vi "LogGrapher.vi"() -> ()   [LabVIEW 2016]
uses:
  <vilib>/regexp/Match Regular Expression.xnode
panel:
  in  "indexes":T1={"angle"=9, "left encoder"=12, "right encoder"=13}
  in  "PlaySpeed":dbl(ring)=1.0 items=["x8"=8.0, "x4"=4.0, "x2"=2.0, "x1"=1.0, "x1/2"=0.5]
  in  "Slide":dbl(slide) scale=0.0..150.0
  out "Robot Tracker":cluster{dbl, dbl}[](graph)
  in  "Play/Pause":enum32{"Play", "Pause"}(radio)=enum."Pause"
  out "Legend":string
  out "Log Grapher":cluster{dbl[], dbl[]}[](graph)
  in  "Log Columns":cluster{"Show":bool, "Data":string}[](array[cluster])
  in  "Column of Time":u32
  in  "Row of Headers":u32=4
  in  "1st Row of Data":u32=5
  in  "Log File Path":path
  # "Enter -1 if not applicable."
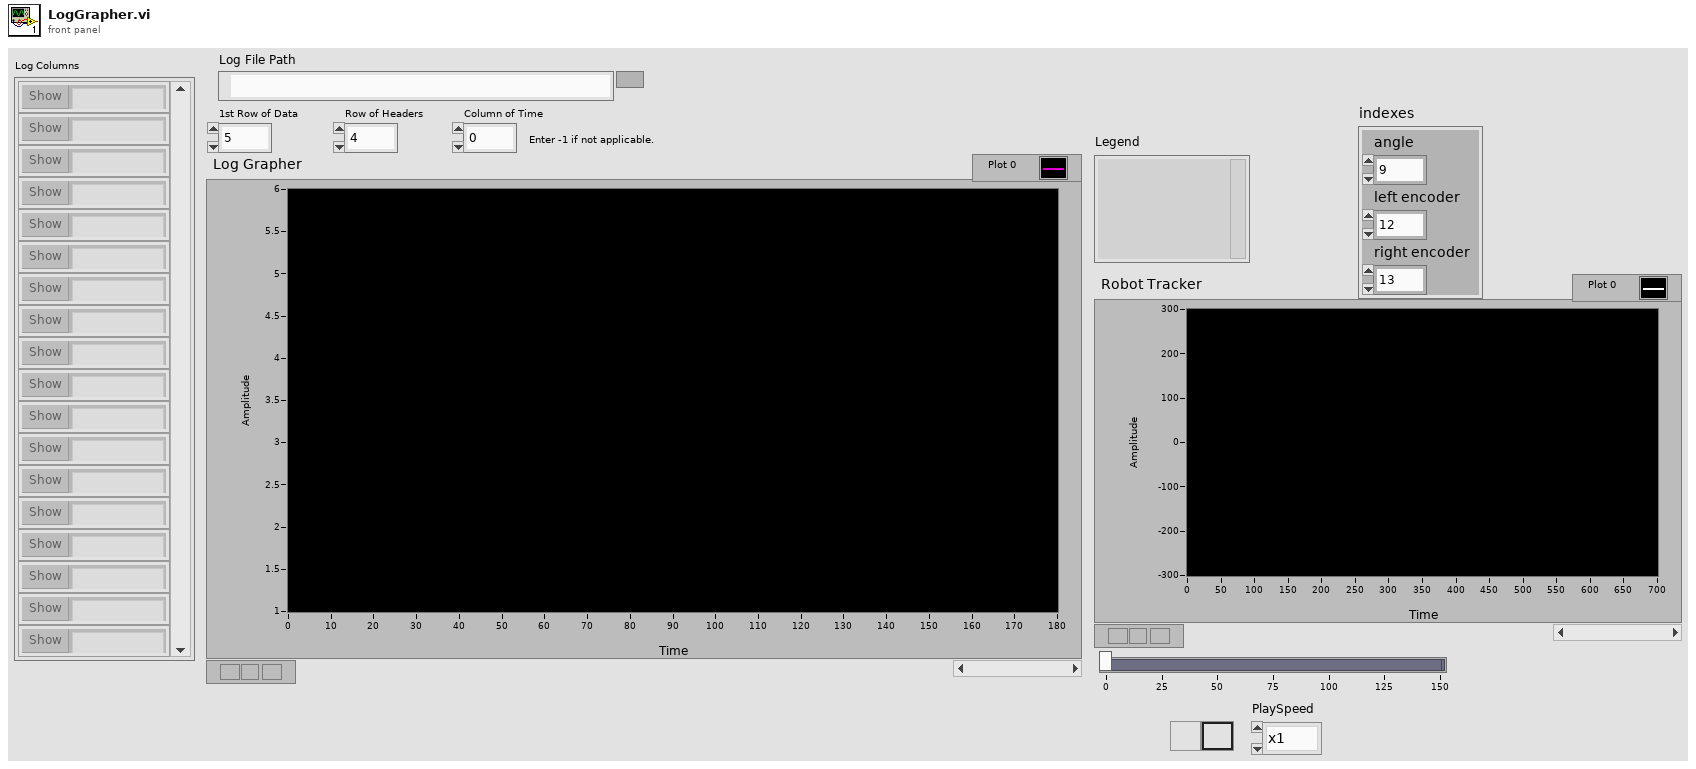
[diagram p1: front panel]
types:
  T1 = cluster{"angle":i32, "left encoder":i32, "right encoder":i32}
  T2 = cluster{"time":i32, "angle":dbl, "left dist":dbl, "right dist":dbl}
  T3 = typedef "LVRangeTypeDef.ctl" = cluster{"Minimum":dbl, "Maximum":dbl, "Increment":dbl, "Minor Increment":dbl, "Start":dbl}
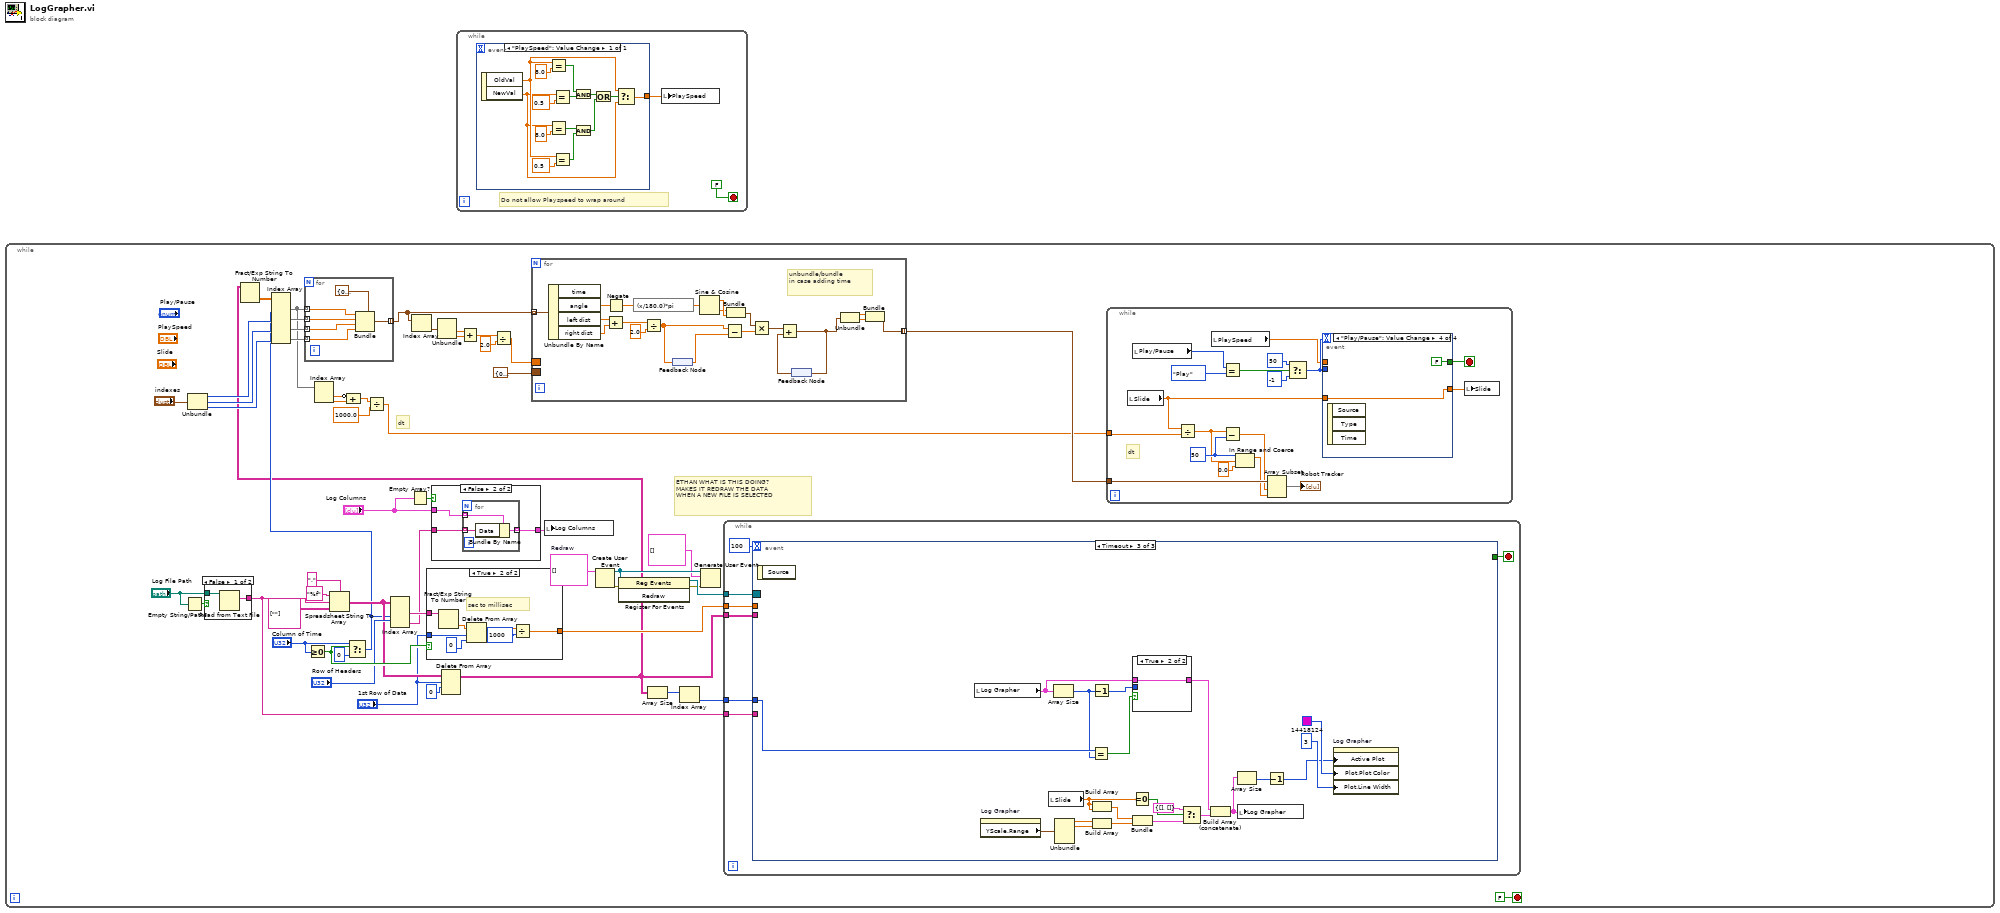
[diagram p0: block diagram]
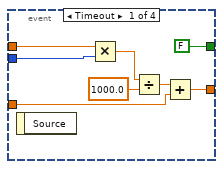
[diagram p2: hidden frame]
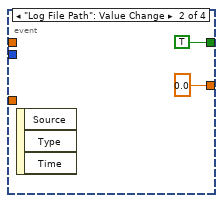
[diagram p3: hidden frame]
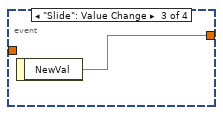
[diagram p4: hidden frame]
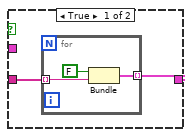
[diagram p5: hidden frame]
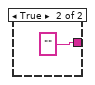
[diagram p6: hidden frame]
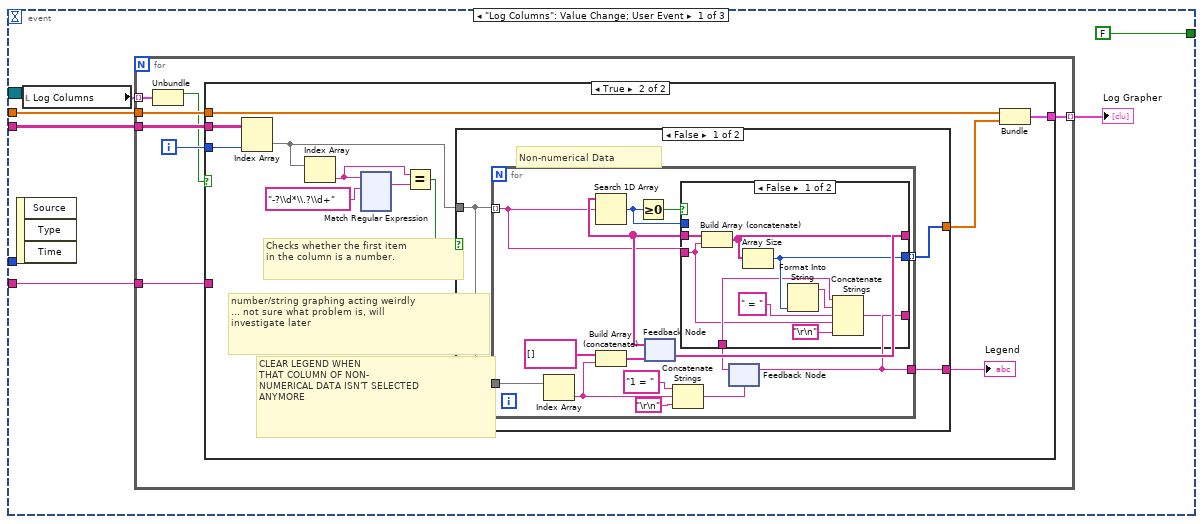
[diagram p7: hidden frame]
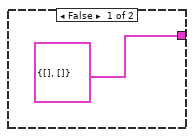
[diagram p8: hidden frame]
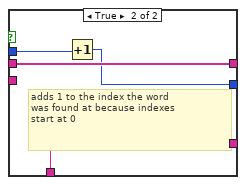
[diagram p9: hidden frame]
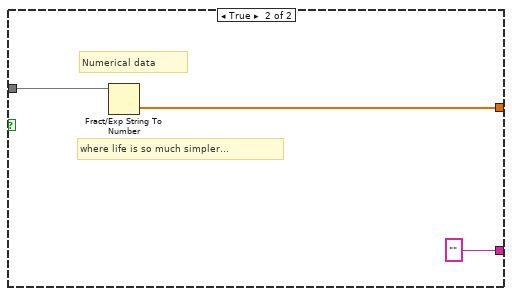
[diagram p10: hidden frame]
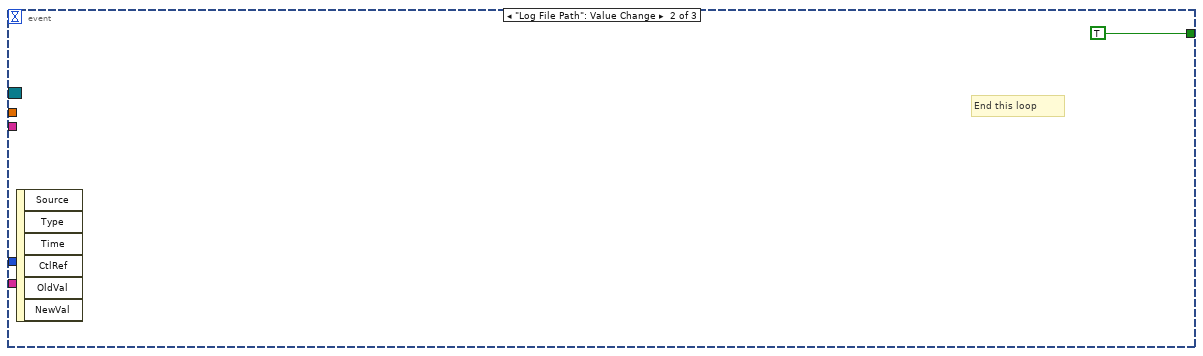
[diagram p11: hidden frame]
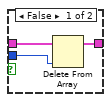
[diagram p12: hidden frame]
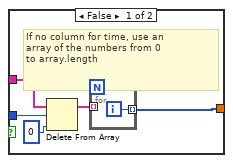
[diagram p13: hidden frame]
diagram:
  n1 = while {
    stop <- FALSE stop-if-true
    w34 = cluster{"Show":bool, "Data":string}[] []  # Redraw
    # "dt"
    # "ETHAN WHAT IS THIS DOING?\nMAKES IT REDRAW THE DATA\nWHEN A NEW FILE IS SELECTED"
    n2 = Empty String/Path?(string/path="Log File Path") -> (empty?=w41:bool)
    n3 = Unbundle("indexes") -> ("angle"=w13:i32, "left encoder"=w12:i32, "right encoder"=w11:i32)
    n4 = case shown="False" w41 {
      tunnel: [w123 ""] -> w28
      tunnel: "Log File Path" -> [w122 _]
      frame False {
        n5 = Read from Text File(file (use dialog)=w122) -> (text=w123:string)  [unwired: 3 in, 3 out]
      }
      frame True {
      }
    }
    n6 = Greater Or Equal To 0?(x="Column of Time") -> (x >= 0?=w47:bool)
    n7 = Spreadsheet String To Array(delimiter (Tab)=",", format string="%f", spreadsheet string=w28, array type (2D Dbl)=string[][] [[""]]) -> (array=w43:string[][])
    n8 = Select(t="Column of Time", s=w47, f=u32 0) -> (s? t:f=w10:u32)
    n9 = Index Array(array=w43, index (col) #1=w10, index (row) #2="Row of Headers") -> (element #1=w50:string[], element #2=w39:string[])  [unwired: 2 in]
    n10 = Empty Array?(array="Log Columns") -> (empty?=w38:bool)
    n11 = case shown="True" w47 {
      tunnel: [w335 w341] -> w36
      tunnel: "1st Row of Data" -> [w332 w340]
      tunnel: w50 -> [w333 w339]
      frame False {
        # "If no column for time, use an\narray of the numbers from 0 \nto array.length"
        n12 = Delete From Array(array=w333, length=w332, index=0) -> (array with subset deleted=w331:string[])  [unwired: 1 out]
        n13 = for {
          tunnel: [w336] -> w335 mode=indexing
          tunnel: w331 -> [_] mode=indexing
          i -> [w336]
        }
      }
      frame True {
        # "sec to millisec"
        n14 = Fract/Exp String To Number(string=w339) -> (number=w338:dbl[])  [unwired: 3 in, 1 out]
        n15 = Delete From Array(array=w338, length=w340, index=0) -> (array with subset deleted=w337:dbl[])  [unwired: 1 out]
        n16 = Divide(x=w337, y=1000) -> (x/y=w341:dbl[])
      }
    }
    n17 = case shown="False" w38 {
      tunnel: [w112 w118] -> w33
      tunnel: w39 -> [w111 w117]
      tunnel: "Log Columns" -> [_ w116]
      frame True {
        n18 = for {
          tunnel: w111 -> [w114] mode=indexing
          tunnel: [w115] -> w112 mode=indexing
          n19 = Bundle(FALSE, "delimiter (Tab)"=w114) -> (w115:cluster{bool, "delimiter (Tab)":string})  [unwired: 1 in]
        }
      }
      frame False {
        n20 = for {
          tunnel: w117 -> [w119] mode=indexing
          tunnel: [w121] -> w118 mode=indexing
          tunnel: w116 -> [w120] mode=indexing
          n21 = Bundle By Name(cluster=w120, "Data"=w119) -> (w121:cluster{"Show":bool, "Data":string})
        }
      }
    }
    n22 = Delete From Array(array=w43, length="1st Row of Data", index (row)=0 ("disabled index (col)")) -> (array with subset deleted=w3:string[][])  [unwired: 1 in, 1 out]
    n23 = Fract/Exp String To Number(string=w3) -> (number=w24:dbl[][])  [unwired: 3 in, 1 out]
    n24 = Index Array(array=w24, index (col) #1=w10, index (col) #2=w13, index (col) #3=w12, index (col) #4=w11) -> (element #1=w9:dbl[], element #2=w27:dbl[], element #3=w26:dbl[], element #4=w25:dbl[])  [unwired: 4 in]
    n25 = for {
      tunnel: w9 -> [w110] mode=indexing
      tunnel: w27 -> [w108] mode=indexing
      tunnel: w26 -> [w107] mode=indexing
      tunnel: w25 -> [w106] mode=indexing
      tunnel: [w105] -> w22 mode=indexing
      n26 = Bundle(cluster=T2 {"time"=0, "angle"=0.0, "left dist"=0.0, "right dist"=0.0}, "time"=w110, "angle"=w108, "left dist"=w107, "right dist"=w106) -> (w105:T2)
    }
    n27 = Index Array(array=w9) -> (element #1=w7:dbl, element #2=w8:dbl)  [unwired: 2 in]
    n28 = Compound Arithmetic op=ADD(invert w7, w8) -> (w6:dbl)
    n29 = Divide(x=w6, y=1000.0) -> (x/y=w4:dbl)
    n30 = Index Array(array=w22) -> (element=w21:T2)  [unwired: 1 in]
    n31 = Unbundle(w21) -> ("left dist"=w18:dbl, "right dist"=w17:dbl)  [unwired: 2 out]
    n32 = Add(x=w18, y=w17) -> (x+y=w19:dbl)
    n33 = Divide(x=w19, y=2.0) -> (x/y=w16:dbl)
    n34 = for {
      tunnel: w22 -> [w104] mode=indexing
      tunnel: [w85] -> w15 mode=indexing
      border: w16 -> [_]
      border: cluster{dbl, dbl} {0.0, 0.0} -> [_]
      # "unbundle/bundle\nin case adding time"
      n35 = Unbundle By Name(w104) -> ("angle"=w92:dbl, "left dist"=w100:dbl, "right dist"=w103:dbl)  [unwired: 1 out]
      n36 = Add(x=w100, y=w103) -> (x+y=w102:dbl)
      n37 = Negate(x=w92) -> (-x=w91:dbl)
      n38 = expression code="(x/180.0)*pi" ("degrees to radians")(w91) -> (w99:dbl)
      n39 = Divide(x=w102, y=2.0) -> (x/y=w90:dbl)
      n40 = feedback #1() -> (w89:dbl)
      n41 = feedback-in #1(w90) -> ()
      n42 = Sine & Cosine(0:w99) -> (1:w98:dbl, 2:w97:dbl)
      n43 = Subtract(x=w90, y=w89) -> (x-y=w95:dbl)
      n44 = Bundle(w97, w98) -> (w96:cluster{dbl, dbl})  [unwired: 1 in]
      n45 = Multiply(x=w96, y=w95) -> (x*y=w94:cluster{dbl, dbl})
      n46 = feedback #2() -> (w93:cluster{dbl, dbl})
      n47 = Add(x=w94, y=w93) -> (x+y=w88:cluster{dbl, dbl})
      n48 = feedback-in #2(w88) -> ()
      n49 = Unbundle(w88) -> (w86:dbl, w87:dbl)
      n50 = Bundle(w86, w87) -> (w85:cluster{dbl, dbl})  [unwired: 1 in]
    }
    n51 = local write "Log Columns"(w33) -> ()
    n52 = Create User Event(user event datatype=w34) -> (user event=w31:refnum<user-event>, error out=w29:errorcluster)  [unwired: 1 in]
    n53 = register-events(error in=w29, w31) -> (reference out=w35:refnum<event-registration>, error out=w32:errorcluster)  [unwired: 1 in]
    n54 = Array Size(array=w3) -> (size(s)=w2:i32[])
    n55 = Index Array(array=w2) -> (element=w1:i32)  [unwired: 1 in]
    n56 = Generate User Event(user event=w31, event data cluster=cluster{"Show":bool, "Data":string}[] [] ("event data"), error in=w32) -> ()  [unwired: 1 in, 2 out]
    n57 = while {
      tunnel: w3 -> [w131]
      tunnel: w36 -> [w130]
      tunnel: w35 -> [w128]
      tunnel: w28 -> [w127]
      tunnel: w1 -> [w126]
      stop <- w129 stop-if-true
      n58 = event shown="[2] Timeout" {
        selector: w128 -> [_ _ _]
        dyn-events: _ -> [_ _ _]
        timeout: 100 -> [_ _ _]
        tunnel: w131 -> [w137 _ _]
        tunnel: w130 -> [w136 _ _]
        tunnel: [FALSE TRUE _] -> w129
        tunnel: w127 -> [w132 _ _]
        tunnel: w126 -> [_ _ w326]
        event "Log Columns": Value Change; User Event {
          n59 = event-data() -> ()  [unwired: 1 in, 3 out]
          n60 = local read "Log Columns"() -> (w133:cluster{"Show":bool, "Data":string}[])
          n61 = for {
            tunnel: w137 -> [w144]
            tunnel: [w142] -> w135 mode=indexing
            tunnel: w136 -> [w141]
            tunnel: w133 -> [w140] mode=indexing
            tunnel: w132 -> [w139]
            i -> [w143]
            n62 = Unbundle(w140) -> ("Show"=w138:bool)  [unwired: 1 out]
            n63 = case shown="True" w138 {
              tunnel: w143 -> [_ w147]
              tunnel: w144 -> [_ w146]
              tunnel: [cluster{dbl[], dbl[]} {[], []} w152] -> w142
              tunnel: w141 -> [_ w151]
              tunnel: w139 -> [_ _]
              frame False {
              }
              frame True {
                # "number/string graphing acting weirdly\n... not sure what problem is, will\ninvestigate later"
                # "CLEAR LEGEND WHEN\nTHAT COLUMN OF NON-\nNUMERICAL DATA ISN'T SELECTED\nANYMORE"
                # "Checks whether the first item \nin the column is a number."
                n64 = Index Array(array=w146, index (col)=w147) -> (element=w148:string[])  [unwired: 1 in]
                n65 = Index Array(array=w148) -> (element=w155:string)  [unwired: 1 in]
                n66 = xnode "Match Regular Expression"("input string"=w155, "regular expression"="-?\\d*\\.?\\d+" ("search string")) -> ("whole match"=w156:string)  [unwired: 4 in, 4 out]
                n67 = Equal?(x=w155, y=w156) -> (x = y?=w154:bool)
                n68 = case shown="False" w154 {
                  tunnel: w148 -> [w157 w189]
                  tunnel: [w159 w188] -> w150
                  tunnel: [w158 ""] -> w153
                  frame False {
                    # "Non-numerical Data"
                    n69 = for {
                      tunnel: w157 -> [w168] mode=indexing
                      tunnel: w157 -> [w174]
                      tunnel: [w166] -> w159 mode=indexing
                      tunnel: [w161] -> w158
                      n70 = Index Array(array=w174) -> (element=w165:string)  [unwired: 1 in]
                      n71 = Build Array (concatenate)(string[] [], w165) -> (w172:string[])
                      n72 = feedback #3(w172) -> (w169:string[])
                      n73 = Search 1D Array(1D array=w169, element=w168) -> (index of element=w170:i32)  [unwired: 1 in]
                      n74 = Greater Or Equal To 0?(x=w170) -> (x >= 0?=w171:bool)
                      n75 = Concatenate Strings("1 = " ("string"), w165, "\r\n") -> (w163:string)
                      n76 = feedback #4(w163) -> (w162:string)
                      n77 = case shown="False" w171 {
                        tunnel: w170 -> [_ w186]
                        tunnel: w169 -> [w183 w187]
                        tunnel: w168 -> [w178 _]
                        tunnel: [w182 w187] -> w167
                        tunnel: [w180 w185] -> w166
                        tunnel: w162 -> [w179 w184]
                        tunnel: [w175 w184] -> w161
                        frame False {
                          n78 = Build Array (concatenate)(w183, w178) -> (w182:string[])
                          n79 = Array Size(array=w182) -> (size(s)=w180:i32)
                          n80 = Format Into String(w180) -> (resulting string=w181:string)  [unwired: 3 in, 1 out]
                          n81 = Concatenate Strings(w179, w181, " = " ("string"), w178, "\r\n") -> (w175:string)
                        }
                        frame True {
                          # "adds 1 to the index the word\nwas found at because indexes\nstart at 0"
                          n82 = Increment(x=w186) -> (x+1=w185:i32)
                        }
                      }
                      n83 = feedback-in #3(w167) -> ()
                      n84 = feedback-in #4(w161) -> ()
                    }
                  }
                  frame True {
                    # "where life is so much simpler..."
                    # "Numerical data"
                    n85 = Fract/Exp String To Number(string=w189) -> (number=w188:dbl[])  [unwired: 3 in, 1 out]
                  }
                }
                "Legend" <- w153
                n86 = Bundle(w151, w150) -> (w152:cluster{dbl[], dbl[]})  [unwired: 1 in]
              }
            }
          }
          "Log Grapher" <- w135
        }
        event "Log File Path": Value Change {
          # "End this loop"
          n87 = event-data() -> ()  [unwired: 1 in, 6 out]
        }
        event Timeout {
          n88 = event-data() -> ()  [unwired: 1 in, 1 out]
          n89 = local read "Log Grapher"() -> (w314:cluster{dbl[], dbl[]}[])
          n90 = property on="Log Grapher" class="XYGraph (strict)"() -> ("YScale.Range"=w309:T3)  [unwired: 2 in, 2 out]
          n91 = local read "Slide"() -> (w321:dbl)
          n92 = Array Size(array=w314) -> (size(s)=w316:i32)
          n93 = Unbundle(w309) -> ("Minimum"=w319:dbl, "Maximum"=w320:dbl)  [unwired: 3 out]
          n94 = Equal?(x=w326, y=w316) -> (x = y?=w313:bool)
          n95 = Decrement(x=w316) -> (x-1=w312:i32)
          n96 = Build Array(w321, w321) -> (w317:dbl[])
          n97 = Build Array(w319, w320) -> (w318:dbl[])
          n98 = Equal To 0?(x=w321) -> (x = 0?=w322:bool)
          n99 = case shown="True" w313 {
            tunnel: w314 -> [w329 w330]
            tunnel: [w327 w330] -> w315
            tunnel: w312 -> [w328 _]
            frame False {
              n100 = Delete From Array(array=w329, index=w328) -> (array with subset deleted=w327:cluster{dbl[], dbl[]}[])  [unwired: 1 in, 1 out]
            }
            frame True {
            }
          }
          n101 = Bundle(w317, w318) -> (w324:cluster{dbl[], dbl[]})  [unwired: 1 in]
          n102 = Select(t=cluster{dbl[], dbl[]} {[], []} ("output cluster"), s=w322, f=w324) -> (s? t:f=w325:cluster{dbl[], dbl[]})
          n103 = Build Array (concatenate)(w315, w325) -> (w308:cluster{dbl[], dbl[]}[])
          n104 = Array Size(array=w308) -> (size(s)=w307:i32)
          n105 = local write "Log Grapher"(w308) -> ()
          n106 = Decrement(x=w307) -> (x-1=w306:i32)
          n107 = property on="Log Grapher" class="XYGraph (strict)"("Active Plot"=w306, "Plot.Plot Color"=u32 14418124, "Plot.Line Width"=u8 3) -> ()  [unwired: 2 in, 2 out]
        }
      }
    }
    n108 = while {
      tunnel: w15 -> [w70]
      tunnel: w4 -> [w54]
      stop <- w71 stop-if-true
      w63 = 50 ("length")
      # "dt"
      n109 = local read "Slide"() -> (w59:dbl)
      n110 = local read "Play/Pause"() -> (w57:enum32{"Play", "Pause"})
      n111 = Divide(x=w59, y=w54) -> (x/y=w62:dbl)
      n112 = local read "PlaySpeed"() -> (w56:dbl)
      n113 = Equal?(x=w57, y=enum32{"Play", "Pause"}."Play") -> (x = y?=w68:bool)
      n114 = Subtract(x=w62, y=w63) -> (x-y=w64:dbl)
      n115 = In Range and Coerce(upper limit=w63, x=w62, lower limit=0.0) -> (coerced(x)=w61:dbl)  [unwired: 1 out]
      n116 = Array Subset(array=w70, index=w64, length=w61) -> (→"Robot Tracker":cluster{dbl, dbl}[])
      n117 = Select(t=50, s=w68, f=-1) -> (s? t:f=w65:i32)
      n118 = event shown="[3] \"Play/Pause\": Value Change" {
        selector: _ -> [_ _ _ _]
        dyn-events: _ -> [_ _ _ _]
        timeout: w65 -> [_ _ _ _]
        tunnel: [FALSE TRUE _ FALSE] -> w71
        tunnel: w59 -> [w78 _ _ w83]
        tunnel: [w77 0.0 ("NewVal") w82 w83] -> w58
        tunnel: w65 -> [w76 _ _ _]
        tunnel: w56 -> [w75 _ _ _]
        event Timeout {
          n119 = event-data() -> ()  [unwired: 1 in, 1 out]
          n120 = Multiply(x=w75, y=w76) -> (x*y=w74:dbl)
          n121 = Divide(x=w74, y=1000.0) -> (x/y=w72:dbl)
          n122 = Add(x=w72, y=w78) -> (x+y=w77:dbl)
        }
        event "Log File Path": Value Change {
          n123 = event-data() -> ()  [unwired: 1 in, 3 out]
        }
        event "Slide": Value Change {
          n124 = event-data() -> ("NewVal"=w82:dbl)  [unwired: 1 in]
        }
        event "Play/Pause": Value Change {
          n125 = event-data() -> ()  [unwired: 1 in, 3 out]
        }
      }
      n126 = local write "Slide"(w58) -> ()
    }
  }
  n127 = while {
    stop <- FALSE stop-if-true
    # "Do not allow Playspeed to wrap around"
    n128 = event shown="[0] \"PlaySpeed\": Value Change" {
      selector: _ -> [_]
      dyn-events: _ -> [_]
      timeout: _ -> [_]
      tunnel: [w355] -> w344
      event "PlaySpeed": Value Change {
        n129 = event-data() -> ("OldVal"=w353:dbl, "NewVal"=w351:dbl)  [unwired: 1 in]
        n130 = Equal?(x=w353, y=8.0) -> (x = y?=w357:bool)
        n131 = Equal?(x=w351, y=8.0) -> (x = y?=w349:bool)
        n132 = Equal?(x=w351, y=0.5) -> (x = y?=w356:bool)
        n133 = Equal?(x=w353, y=0.5) -> (x = y?=w350:bool)
        n134 = And(x=w357, y=w356) -> (x .and. y?=w348:bool)
        n135 = And(x=w349, y=w350) -> (x .and. y?=w347:bool)
        n136 = Or(x=w348, y=w347) -> (x .or. y?=w346:bool)
        n137 = Select(t=w353, s=w346, f=w351) -> (s? t:f=w355:dbl)
      }
    }
    n138 = local write "PlaySpeed"(w344) -> ()
  }
